vi "Sin9225-7_FPGA.vi"(1 "x [pi]":fxp<+/-,40,5>) -> (0 "sin(x)":fxp<+/-,36,2>)   [LabVIEW 2021]
uses:
  <vilib>/rvi/FXPMathLib/FxpSinAndCos/subVIs/nifxpmath_SinAndCos_SimConfig.ctl
  <vilib>/rvi/FXPMathLib/FxpSinAndCos/simVIs/DllFxpSinAndCosTemp_sub.vi
  <vilib>/rvi/FXPMathLib/FxpSinAndCos/XNode/nifxpmath_SinAndCos.xnode
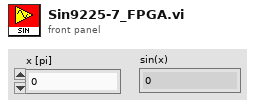
[diagram p1: front panel]
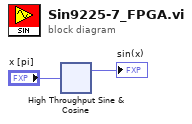
[diagram p0: block diagram]
diagram:
  n1 = xnode "High Throughput Sine & Cosine"("x (pi)"="x [pi]") -> ("sin(x)"=→"sin(x)":fxp<+/-,36,2>)  [unwired: 1 out]
